vi "First Step.vi"(8 "error in (no error)":errorcluster, 11 "Wavelength Digikröm.lvclass in":refnum<class "Wavelength Digikröm.lvclass">) -> (0 "error out":errorcluster, 2 "Current Position":dbl, 3 "Wavelength Digikröm.lvclass out":refnum<class "Wavelength Digikröm.lvclass">)   [LabVIEW 2023, in "Wavelength Digikröm.lvclass"]
doc: "Goto step #0 - the first step. If desired, the scanner may do this in a different way than usual (i.e. by preparing to move a long distance, or reset to home position.)"
uses:
  Scanner/Scanner.lvclass
  Instruments/Utility Classes/Scannable/Scannable.lvclass
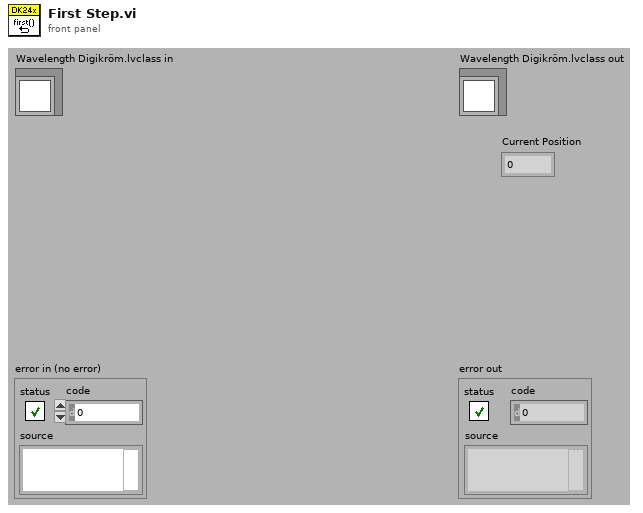
[diagram p1: front panel]
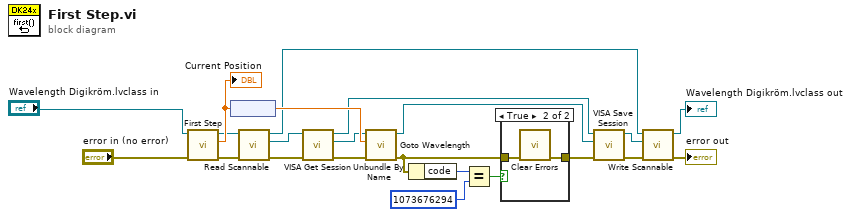
[diagram p0: block diagram]
diagram:
  n1 = call-parent "First Step.vi"("error in (no error)"="error in (no error)", "Scanner.lvclass in"="Wavelength Digikröm.lvclass in") -> ("error out"=w10:errorcluster, "Current Position"=w20:dbl, "Scanner.lvclass out"=w14:refnum<class "Wavelength Digikröm.lvclass">)  [unwired: 7 out]
  "Current Position" <- w20
  n2 = node(w20) -> (w19:dbl[unit])
  n3 = call-dynamic "Read Scannable.vi"("error in (no error)"=w10, "Scanner.lvclass in"=w14) -> ("error out"=w9:errorcluster, "Scannable.lvclass"=w13:refnum<class "Scannable.lvclass">, "Scanner.lvclass out"=w3:refnum<class "Wavelength Digikröm.lvclass">)  [unwired: 7 out]
  n4 = call-dynamic "VISA Get Session.vi"("error in (no error)"=w9, "Instrument.lvclass in"=w13) -> ("error out"=w8:errorcluster, "VISA Resource Name"=w12:refnum<visa-resource-name>, "Instrument.lvclass out"=w1:refnum<class "Scannable.lvclass">)  [unwired: 7 out]
  n5 = call "Goto Wavelength.vi"("error in (no error)"=w8, "WAVELENGTH"=w19, "VISA resource name"=w12) -> ("error out"=w18:errorcluster, "VISA resource name out"=w11:refnum<visa-resource-name>)  [unwired: 7 out]
  n6 = Unbundle By Name(w18) -> ("code"=w16:i32)
  n7 = Equal?(x=w16, y=1073676294) -> (x = y?=w15:bool)
  n8 = case shown="True" w15 {
    tunnel: w18 -> [w23 w25]
    tunnel: [w23 w24] -> w7
    frame False {
    }
    frame True {
      n9 = call <vilib>:"Clear Errors.vi"("error in (no error)"=w25) -> ("error out"=w24:errorcluster)  [unwired: 5 in, 1 out]
    }
  }
  n10 = call-dynamic "VISA Save Session.vi"("error in (no error)"=w7, "VISA Resource Name"=w11, "Instrument.lvclass in"=w1) -> ("error out"=w6:errorcluster, "Instrument.lvclass out"=w2:refnum<class "Scannable.lvclass">)  [unwired: 7 out]
  n11 = call-dynamic "Write Scannable.vi"("error in (no error)"=w6, "Scannable.lvclass"=w2, "Scanner.lvclass in"=w3) -> ("error out"=→"error out":errorcluster, "Scanner.lvclass out"=→"Wavelength Digikröm.lvclass out":refnum<class "Wavelength Digikröm.lvclass">)  [unwired: 7 out]
